vi "Parse Burst Length.vi"(8 "error in (no error)":errorcluster, 11 "Burst Length in":string) -> (0 "error out":errorcluster, 3 "BurstLength":T1)   [LabVIEW 2018, in "Config Parser BML.lvlib" / "Config Parser BML.lvclass"]
uses:
  Config Parser BML.lvclass
  Ctls/Burst Length.ctl
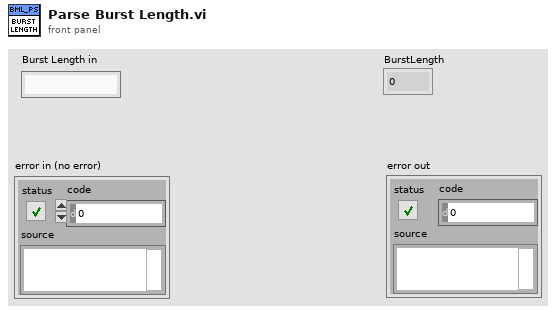
[diagram p1: front panel]
types:
  T1 = typedef "Burst Length.ctl" = enum8{"0", "2", "3", "4", "5", "8", "16", "32"}
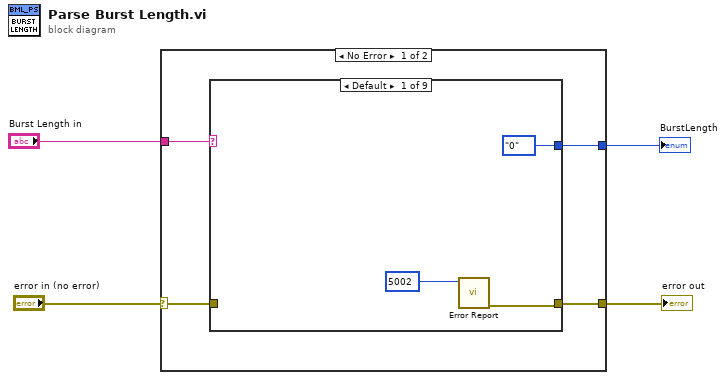
[diagram p0: block diagram]
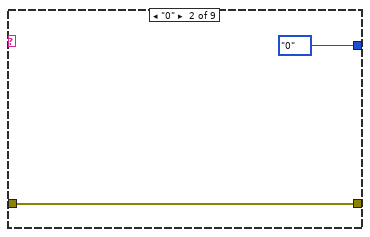
[diagram p2: hidden frame]
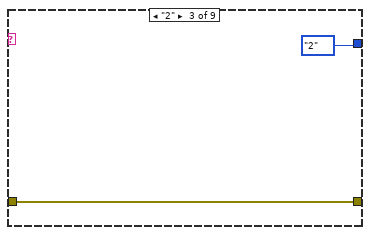
[diagram p3: hidden frame]
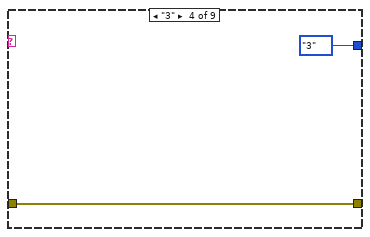
[diagram p4: hidden frame]
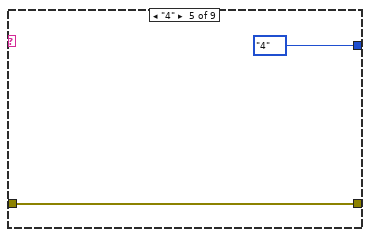
[diagram p5: hidden frame]
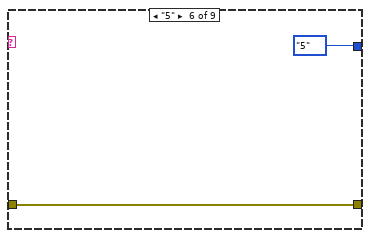
[diagram p6: hidden frame]
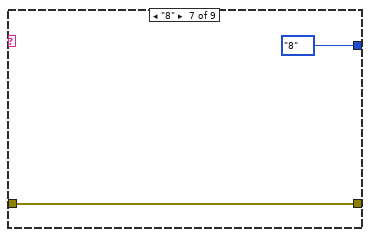
[diagram p7: hidden frame]
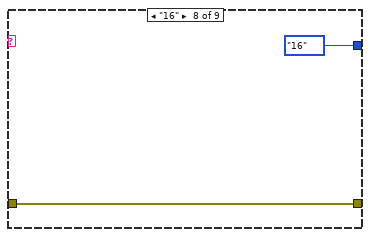
[diagram p8: hidden frame]
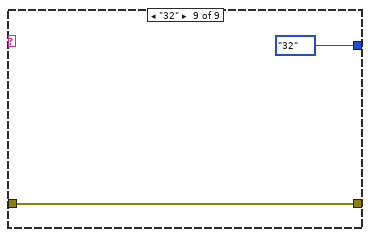
[diagram p9: hidden frame]
diagram:
  n1 = case shown="No Error" "error in (no error)" {
    selector: "error in (no error)" -> [w8 w28]
    tunnel: "Burst Length in" -> [w7 _]
    tunnel: [w6 w28] -> w2
    tunnel: [w5 _] -> w1
    frame No Error {
      n2 = case shown="Default" w7 {
        tunnel: w8 -> [_ w13 w15 w17 w19 w21 w23 w25 w27]
        tunnel: [w9 w13 w15 w17 w19 w21 w23 w25 w27] -> w6
        tunnel: [Burst_Length."0" ("BurstLength") Burst_Length."0" ("BurstLength") Burst_Length."2" ("BurstLength") Burst_Length."3" ("BurstLength") Burst_Length."4" ("BurstLength") Burst_Length."5" ("BurstLength") Burst_Length."8" ("BurstLength") Burst_Length."16" ("BurstLength") Burst_Length."32" ("BurstLength")] -> w5
        frame Default {
          n3 = call "Error Report.vi"("Error Code"=i16 5002) -> ("error out"=w9:errorcluster)  [unwired: 10 in]
        }
        frame "0" {
        }
        frame "2" {
        }
        frame "3" {
        }
        frame "4" {
        }
        frame "5" {
        }
        frame "8" {
        }
        frame "16" {
        }
        frame "32" {
        }
      }
    }
    frame Error {
    }
  }
  "error out" <- w2
  "BurstLength" <- w1
